vi "Delete Tree.vi"(7 "Tree ID":string, 8 "Error In":errorcluster, 11 "Tree Manager":refnum<data-value>) -> (0 "Error Out":errorcluster, 3 "Tree Manager":refnum<data-value>)   [LabVIEW 2017, in "Tree API.lvlib" / "Tree.lvclass"]
doc: "Delete Tree and all its children. \n\nIf any of the deleted Trees contained attributes of Tree Data.lvclass data type, those attributes will be realeased with the Release.vi dynamically dispatched method.\n\nFor safety purposes this uses not only the specified Tree Data types but all Tree Data types that match from memory."
uses:
  Tree.lvclass
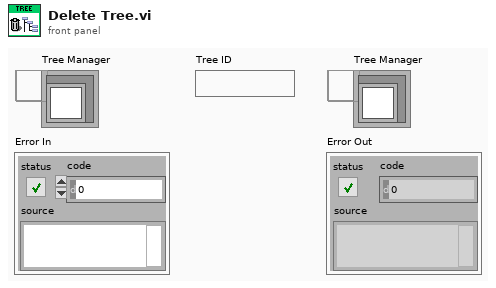
[diagram p1: front panel]
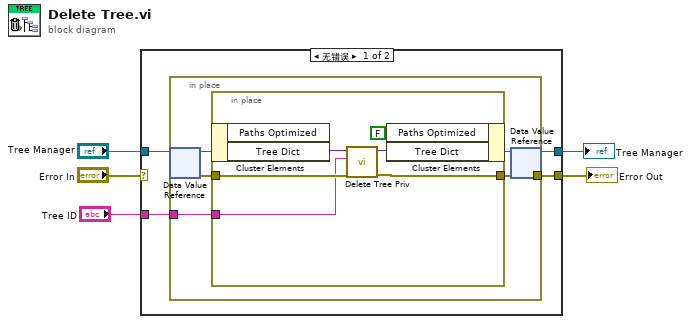
[diagram p0: block diagram]
diagram:
  n1 = case shown="无错误" "Error In" {
    selector: "Error In" -> [_ w21]
    tunnel: "Tree Manager" -> [w9 w22]
    tunnel: [w8 w22] -> w4
    tunnel: [w7 w21] -> w2
    tunnel: "Tree ID" -> [w6 _]
    frame No Error {
      n2 = in-place {
        in-place-border: [w13] -> w7
        in-place-border: w6 -> [w10]
        n3 = in-place-dvr #1(w9) -> (w14:refnum<class "Tree.lvclass">, w11:errorcluster)
        n4 = in-place {
          in-place-border: [w17] -> w13
          in-place-border: w11 -> [w18]
          in-place-border: w10 -> [w16]
          n5 = in-place-cluster #2(w14) -> ("Tree Dict"=w20:variant)  [unwired: 1 out]
          n6 = call "Delete Tree Priv.vi"("Error In"=w18, "Unique ID"=w16, "Tree Dictionary In"=w20) -> ("Error Out"=w17:errorcluster, "Tree Dictionary Out"=w19:variant)  [unwired: 7 in]
          n7 = in-place-cluster #2("Paths Optimized"=FALSE, "Tree Dict"=w19) -> (w12:refnum<class "Tree.lvclass">)
        }
        n8 = in-place-dvr #1(w12) -> (w8:refnum<data-value>)  [unwired: 1 out]
      }
    }
    frame Error {
    }
  }
  "Tree Manager" <- w4
  "Error Out" <- w2
